vi "Tmp_M Initialize.vi"(8 "error in (no error)":errorcluster, 11 "VISA Refnum in":refnum<visa-resource-name>) -> (0 "error out":errorcluster, 2 "TM Revision":T1, 3 "VISA Refnum out":refnum<visa-resource-name>)   [LabVIEW 2024, in "Magnet module.lvlib"]
doc: "Initialize comunication with Temperature Monitor and gets its revision info. At least model name should be send as message to master module."
uses:
  Magnet module.lvlib
  ctl/TM Revision.ctl
  <vilib>/Instr/_visa.llb/VISA Configure Serial Port (Instr).vi
  <instrlib>/Lake Shore Cryotronics 218/Lake Shore Cryotronics 218.lvlib
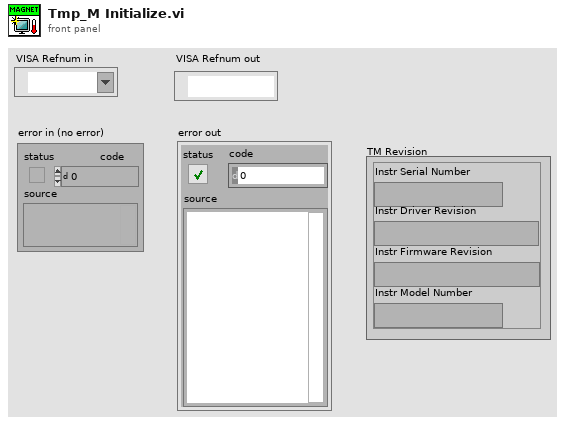
[diagram p1: front panel]
types:
  T1 = typedef "Magnet module.lvlib/TM Revision.ctl" = cluster{"Instr Serial Number":string, "Instr Driver Revision":string, "Instr Firmware Revision":string, "Instr Model Number":string}
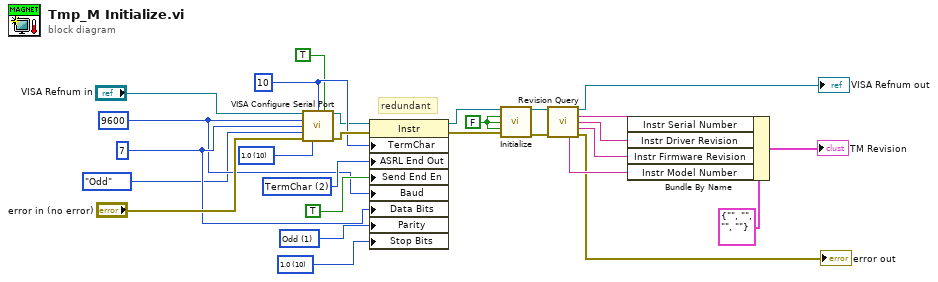
[diagram p0: block diagram]
diagram:
  w1 = u16 10 items=["1.0"=10, "1.5"=15, "2.0"=20] ("Serial Settings:Stop Bits")
  w2 = u16 1 items=["None", "Odd", "Even", "Mark", "Space"] ("Serial Settings:Parity")
  w18 = FALSE
  w24 = u16 2 items=["None", "Last Bit", "TermChar", "Break"] ("Serial Settings:End Mode for Writes")
  w5 = u16 7 ("data bits (8)")
  w4 = u32 9600 ("baud rate (9600)")
  w21 = u16 10 items=["1.0"=10, "1.5"=15, "2.0"=20] ("stop bits (10: 1 bit)")
  w23 = u8 10 ("termination char\n(0xA = '\\n' = LF)")
  # "redundant"
  n1 = call-poly "VISA Configure Serial Port"("VISA resource name"="VISA Refnum in", "termination char\n(0xA = '\\n' = LF)"=w23, "Enable Termination\nChar (T)"=TRUE ("Enable Termination\nChar (T)"), "baud rate (9600)"=w4, "data bits (8)"=w5, "parity (0:none)"=enum16{"None", "Odd", "Even", "Mark", "Space"}."Odd", "error in (no error)"="error in (no error)", "stop bits (10: 1 bit)"=w21) -> ("VISA resource name out"=w19:refnum<visa-resource-name>, "error out"=w26:errorcluster)  [unwired: 6 in]
  n2 = property class="Instr"(reference=w19, error in=w26, "TermChar"=w23, "ASRL End Out"=w24, "Send End En"=TRUE ("Message Based Settings:Send End Enable"), "Baud"=w4, "Data Bits"=w5, "Parity"=w2, "Stop Bits"=w1) -> (reference out=w7:refnum<visa-resource-name>, error out=w8:errorcluster)
  n3 = call <instrlib>:"Initialize.vi"("VISA resource name"=w7, "ID Query (T: Check)"=w18, "Reset (T: Reset)"=w18, "Reset Defaults (F:Dont Reset)"=w18, "error in (no error)"=w8) -> ("VISA resource name out"=w9:refnum<visa-resource-name>, "error out"=w10:errorcluster)  [unwired: 9 in]
  n4 = call <instrlib>:"Revision Query.vi"("VISA resource name"=w9, "error in (no error)"=w10) -> ("VISA resource name out"=→"VISA Refnum out":refnum<visa-resource-name>, "Instr Serial Number"=w14:string, "Instr Driver Revision"=w15:string, "Instr Firmware Revision"=w16:string, "Instr Model Number"=w17:string, "error out"=→"error out":errorcluster)  [unwired: 8 in]
  n5 = Bundle By Name(cluster=T1 {"Instr Serial Number"="", "Instr Driver Revision"="", "Instr Firmware Revision"="", "Instr Model Number"=""} ("Revision"), "Instr Serial Number"=w14, "Instr Driver Revision"=w15, "Instr Firmware Revision"=w16, "Instr Model Number"=w17) -> (→"TM Revision":T1)
